vi "STICK_house_debugOnly.vi"() -> ()   [LabVIEW 2014]
panel:
  out "P2":T1
  out "P1":T2
  out "?":bool
  out "?":bool
  out "?":bool
  out "?":bool
  out "?":bool
  out "?":bool
  out "?":bool
  out "?":bool
  out "?":bool
  out "?":bool
  out "?":bool
  out "?":bool
  out "?":bool
  in  "IDA 0 [V]":dbl min=0.0 max=2.0
  out "error out":errorcluster
  out "8 wire data":u8
  in  "VISA resource name":refnum<visa-resource-name>
  out "Device ID":string
  in  "Stop Button":bool
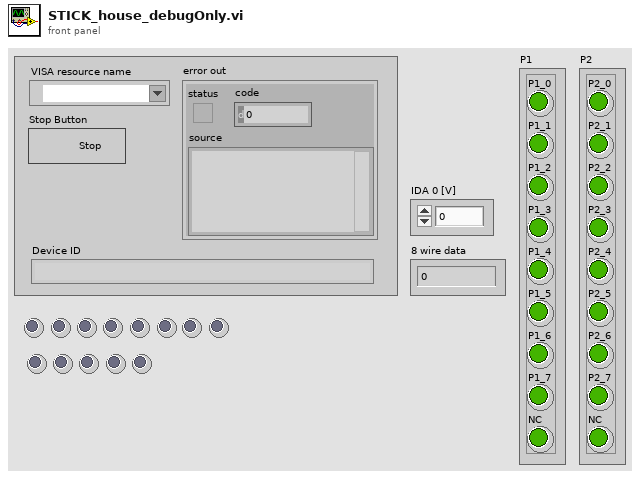
[diagram p1: front panel]
types:
  T1 = cluster{"P2_0":bool, "P2_1":bool, "P2_2":bool, "P2_3":bool, "P2_4":bool, "P2_5":bool, "P2_6":bool, "P2_7":bool, "NC":bool}
  T2 = cluster{"P1_0":bool, "P1_1":bool, "P1_2":bool, "P1_3":bool, "P1_4":bool, "P1_5":bool, "P1_6":bool, "P1_7":bool, "NC":bool}
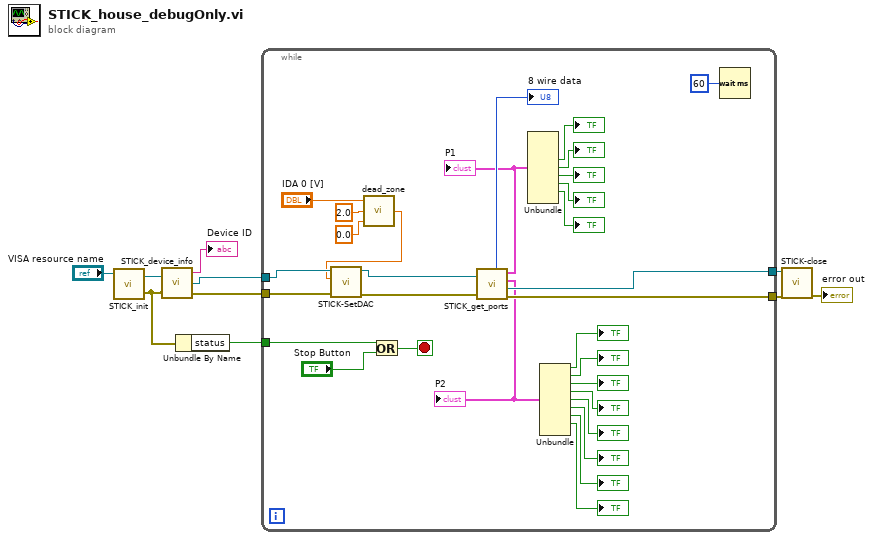
[diagram p0: block diagram]
diagram:
  n1 = call "STICK_init.vi"("VISA Refnum in"="VISA resource name") -> ("error out"=w5:errorcluster, "VISA Refnum out"=w6:refnum<visa-resource-name>)  [unwired: 1 in]
  n2 = call "STICK_device_info.vi"("VISA Refnum in"=w6, "error in (no error)"=w5) -> ("read buffer"=→"Device ID":string, "VISA Refnum out"=w3:refnum<visa-resource-name>, "error out"=w4:errorcluster)
  n3 = Unbundle By Name(w5) -> ("status"=w10:bool)
  n4 = while {
    tunnel: w10 -> [w35]
    tunnel: [w36] -> w7
    tunnel: w4 -> [w33]
    tunnel: w3 -> [w34]
    tunnel: [w30] -> w1
    stop <- w39 stop-if-true
    n5 = call "dead_zone.vi"("min"=0.0, "max"=2.0, "number in"="IDA 0 [V]") -> ("number out"=w11:dbl)
    n6 = call "STICK-SetDAC.vi"("error in (no error)"=w33, "IDA 0 [V]"=w11, "VISA resource name"=w34) -> ("error out"=w32:errorcluster, "VISA resource name out"=w31:refnum<visa-resource-name>)  [unwired: 3 in]
    n7 = Or(x=w35, y="Stop Button") -> (x .or. y?=w39:bool)
    n8 = call "STICK_get_ports.vi"("error in (no error)"=w32, "VISA Refnum in"=w31) -> ("error out"=w36:errorcluster, "VISA Refnum out"=w30:refnum<visa-resource-name>, "P2"=w23:T1, "P1"=w29:T2, "data"=→"8 wire data":u8)
    "P1" <- w29
    "P2" <- w23
    n9 = Unbundle(w29) -> ("P1_3"=→"?":bool, "P1_4"=→"?":bool, "P1_5"=→"?":bool, "P1_6"=→"?":bool, "P1_7"=→"?":bool)  [unwired: 4 out]
    n10 = Unbundle(w23) -> ("P2_0"=→"?":bool, "P2_1"=→"?":bool, "P2_2"=→"?":bool, "P2_3"=→"?":bool, "P2_4"=→"?":bool, "P2_5"=→"?":bool, "P2_6"=→"?":bool, "P2_7"=→"?":bool)  [unwired: 1 out]
    n11 = Wait (ms)(milliseconds to wait=u32 60) -> ()  [unwired: 1 out]
  }
  n12 = call "STICK-close.vi"("error in (no error)"=w7, "VISA resource name"=w1) -> ("error out"=→"error out":errorcluster)  [unwired: 4 in, 1 out]
